vi "LEDSTest.vi"() -> ()   [LabVIEW 2013]
uses:
  LEDSaction.ctl
panel:
  in  "On/Off":bool
  in  "Type":T1
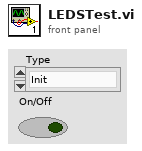
[diagram p1: front panel]
types:
  T1 = typedef "LEDSaction.ctl" = enum16{"Init", "10SecondsLeft", "LimitDown", "LimitUp", "CollectDown", "CollectUp", "NotHot", "Hot", "Shift", "RollBack", "RollFwd", "Shoot", "Distance Low", "DistanceHigh", "PressureLow", "PressureHigh"}
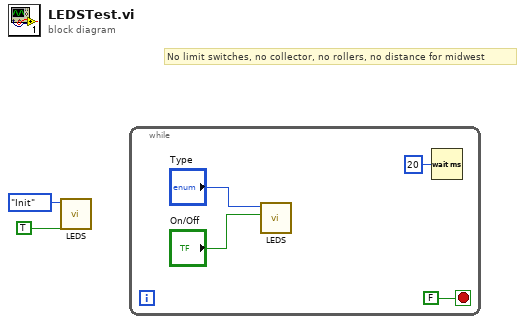
[diagram p0: block diagram]
diagram:
  # "No limit switches, no collector, no rollers, no distance for midwest"
  n1 = call "LEDS.vi"("On/Off"=TRUE, "Type"=LEDSaction."Init") -> ()  [unwired: 9 in, 1 out]
  n2 = while {
    stop <- FALSE stop-if-true
    n3 = call "LEDS.vi"("On/Off"="On/Off", "Type"="Type") -> ()  [unwired: 9 in, 1 out]
    n4 = Wait (ms)(milliseconds to wait=u32 20) -> ()  [unwired: 1 out]
  }
